vi "CRYGet Changed Acquisition Curve Name.vi"(4 "Change Record Curve Name?":bool, 5 "Origin MR0":string[][](array[string]), 6 "Load?":bool, 7 "Change Channels":bool, 8 "Changed Name Table in":string[][](array[string]), 9 "use ch name":bool, 10 "Old Name":string[][](array[string]), 11 "New Name":string[][](array[string])) -> (0 "Changed Name Table  out":string[][](array[string]))   [LabVIEW 2013]
panel:
  out "Changed Name Table in 2":string[][](array[string])
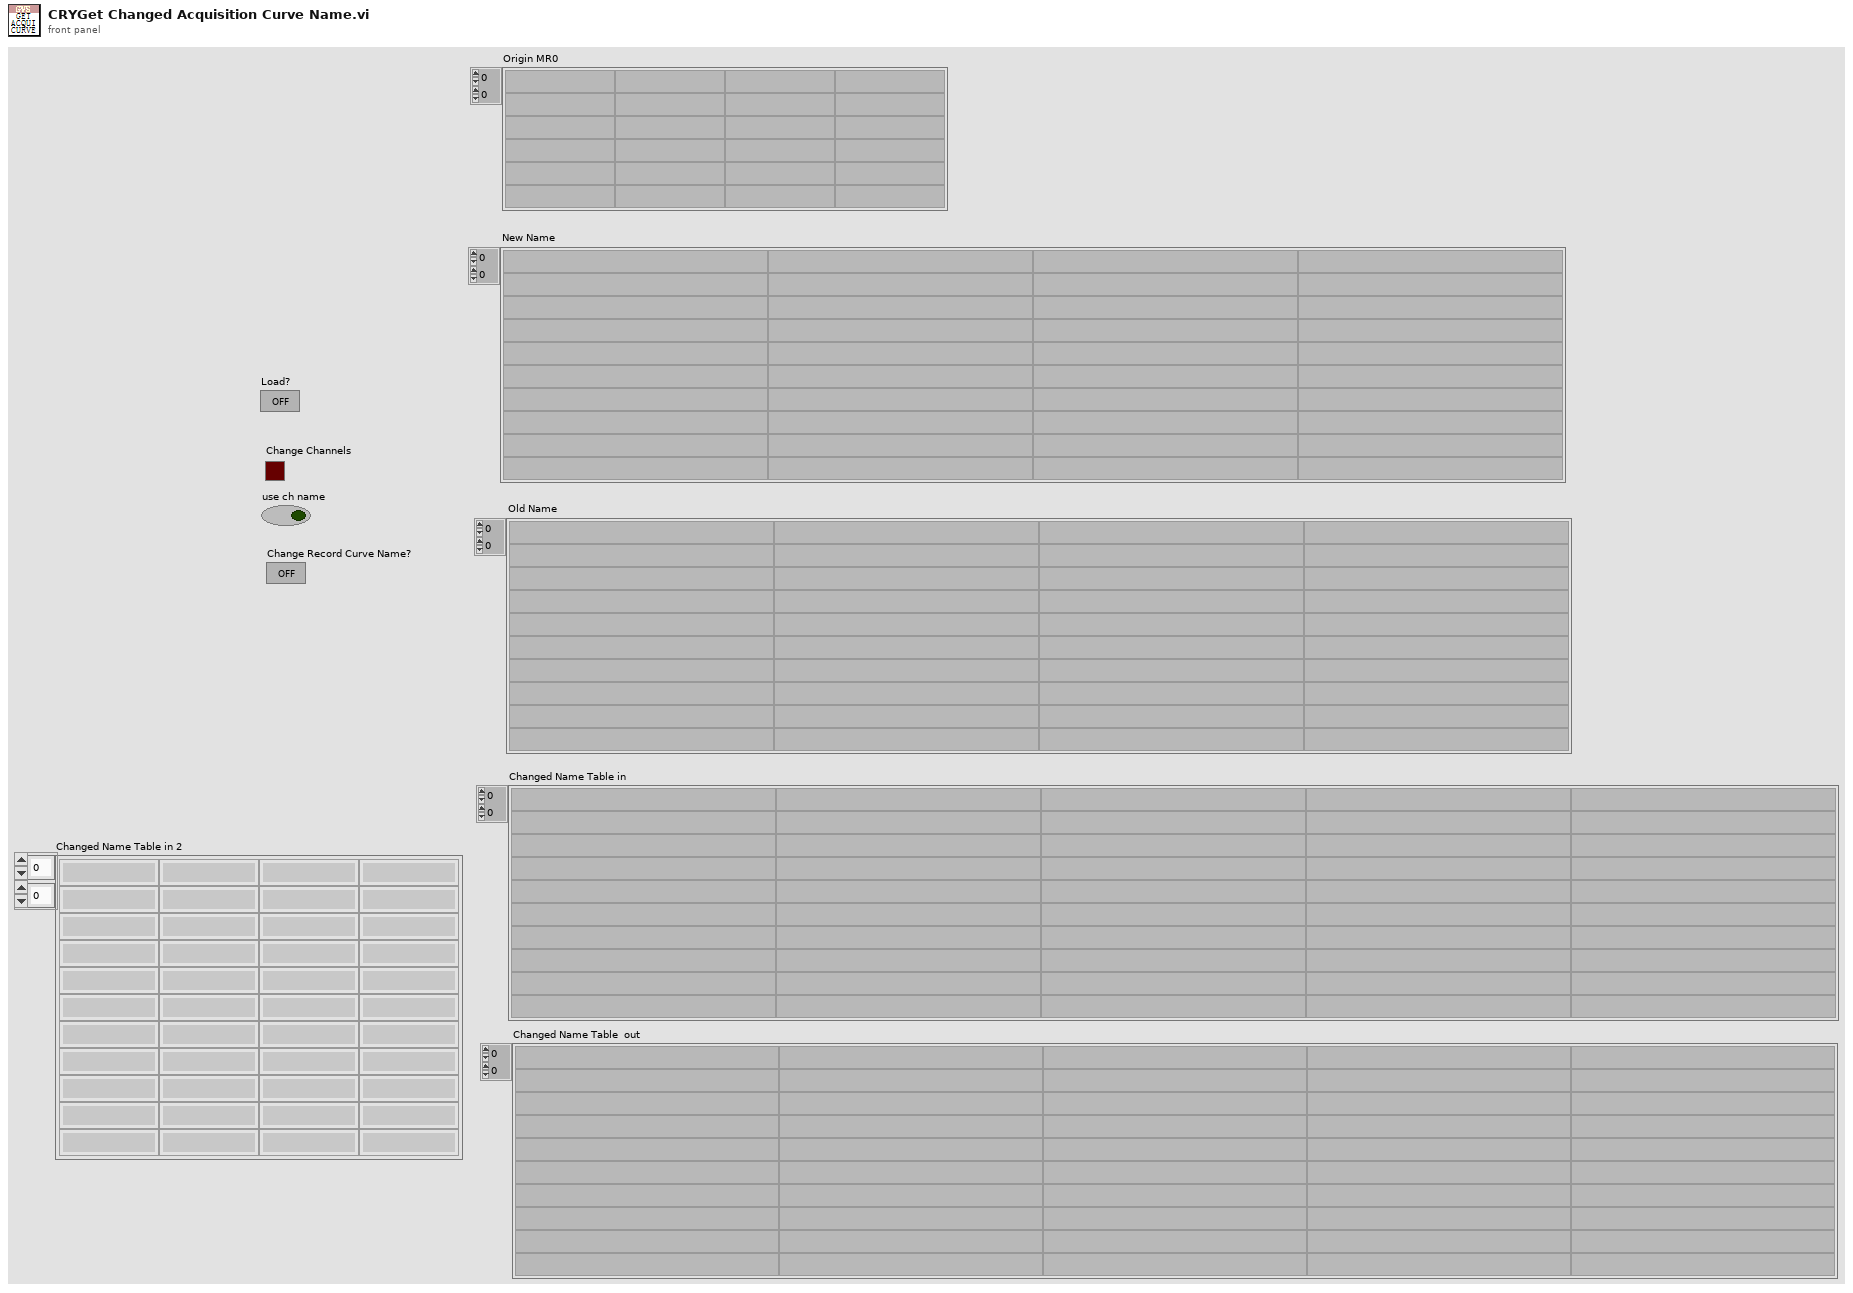
[diagram p1: front panel]
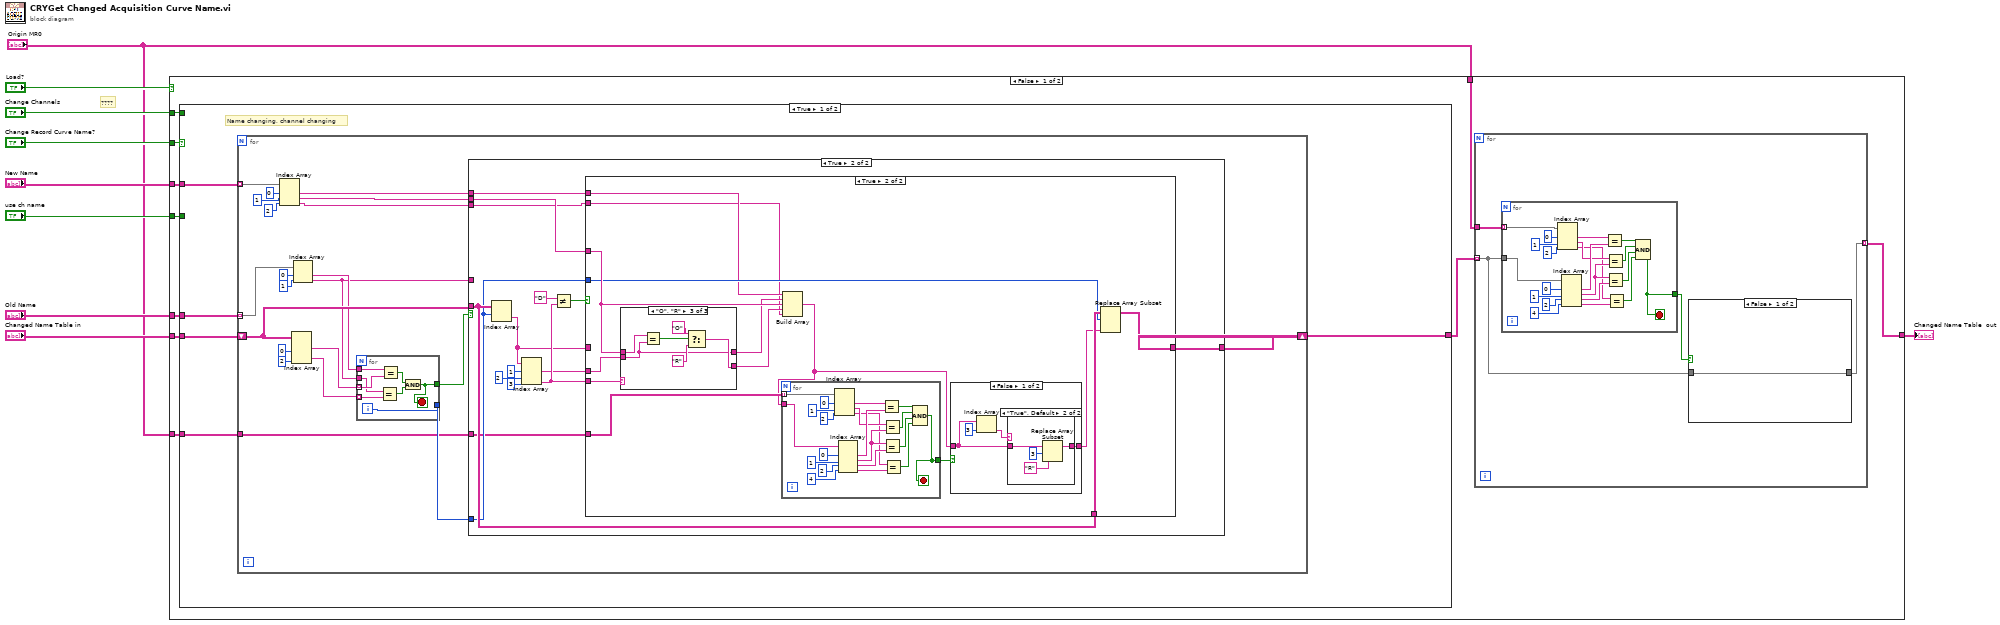
[diagram p0: block diagram]
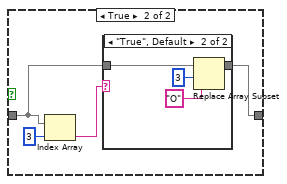
[diagram p2: hidden frame]
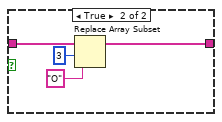
[diagram p7: hidden frame]
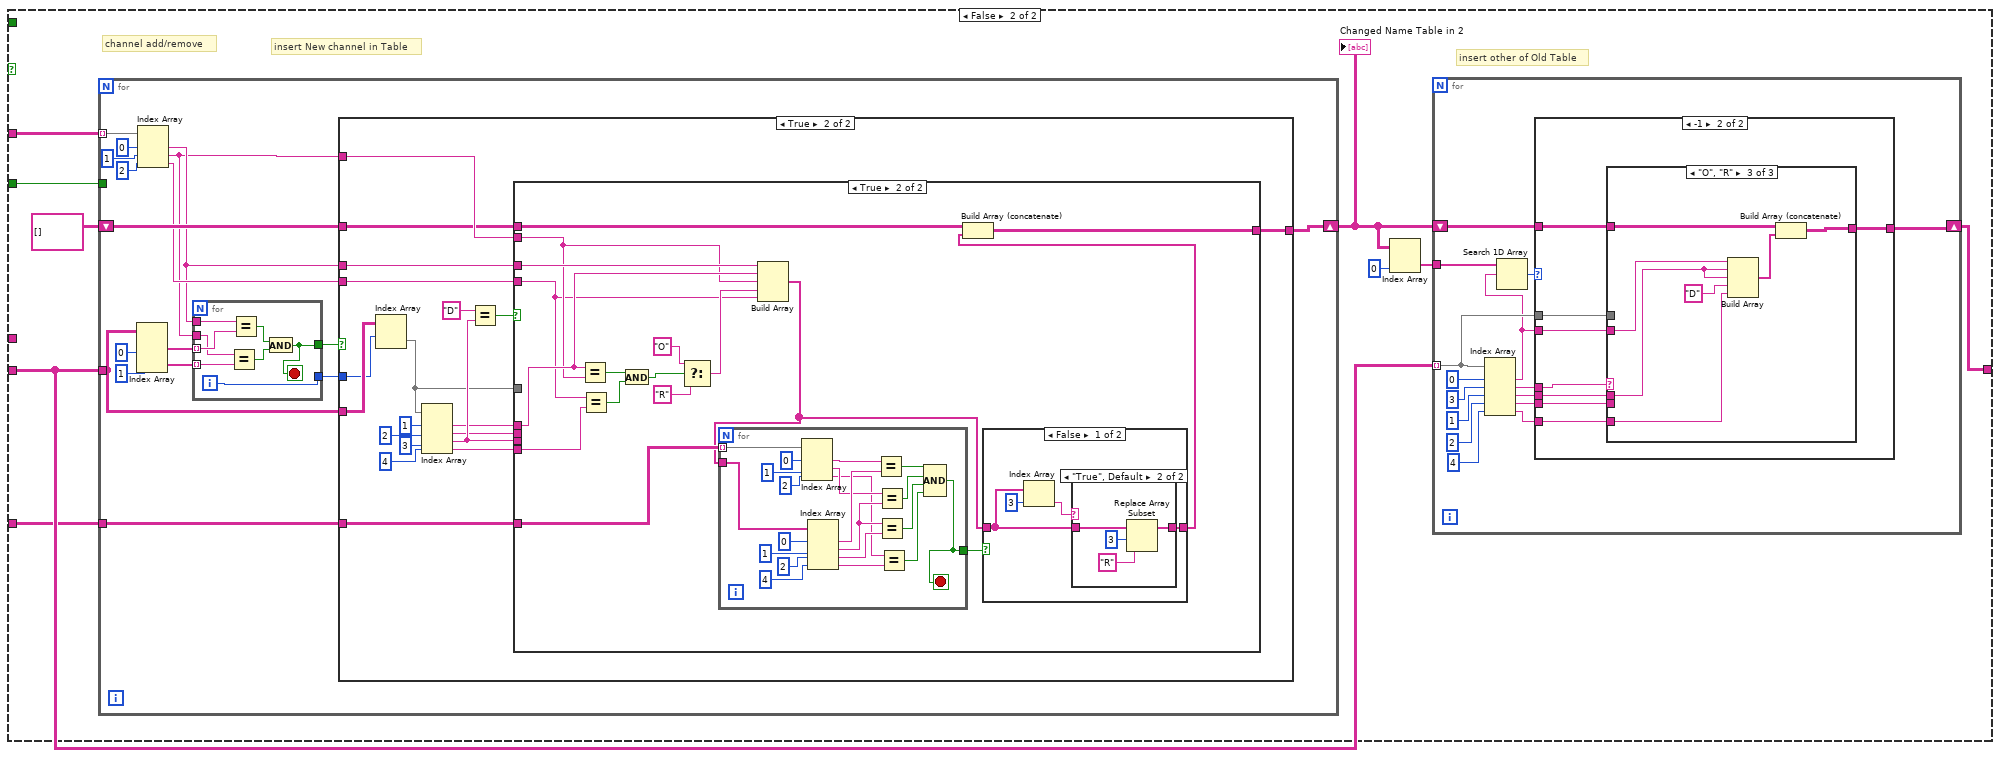
[diagram p10: hidden frame]
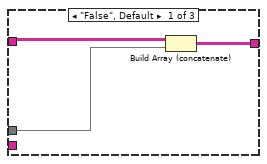
[diagram p12: hidden frame]
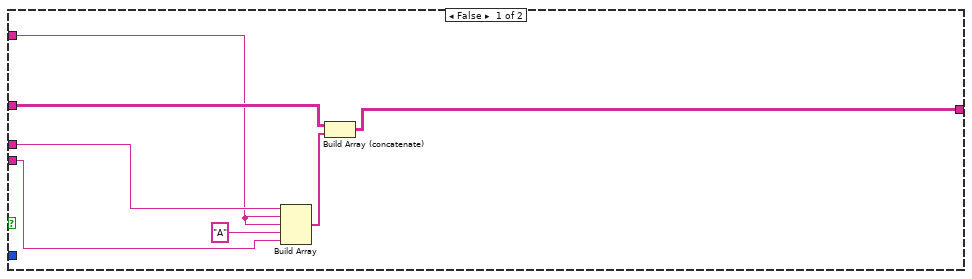
[diagram p14: hidden frame]
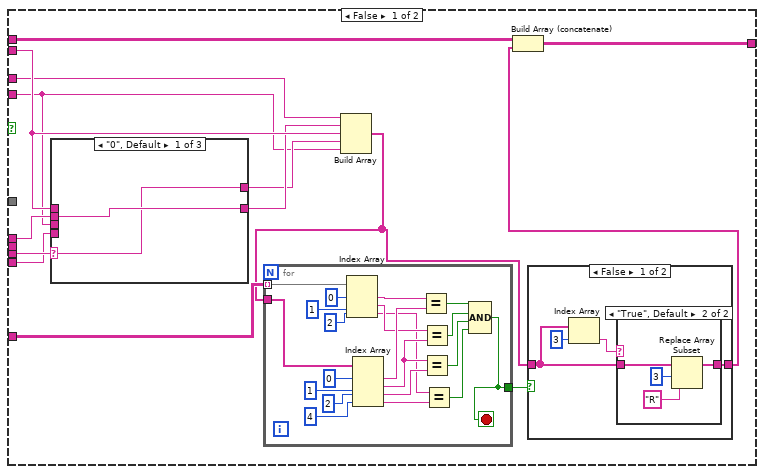
[diagram p15: hidden frame]
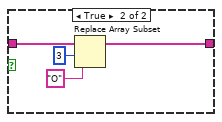
[diagram p17: hidden frame]
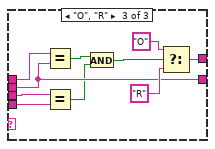
[diagram p19: hidden frame]
diagram:
  # "????"
  n1 = case shown="False" "Load?" {
    tunnel: [w11 w372] -> w9
    tunnel: "Changed Name Table in" -> [w19 _]
    tunnel: "Change Record Curve Name?" -> [w18 _]
    tunnel: "use ch name" -> [w17 _]
    tunnel: "Change Channels" -> [w16 _]
    tunnel: "New Name" -> [w15 w373]
    tunnel: "Old Name" -> [w14 _]
    tunnel: "Origin MR0" -> [w13 _]
    tunnel: "Origin MR0" -> [w10 _]
    frame False {
      n2 = case shown="True" w18 {
        tunnel: [w56 w169] -> w12
        tunnel: w19 -> [w59 w165]
        tunnel: w14 -> [w58 _]
        tunnel: w15 -> [w57 w172]
        tunnel: w17 -> [_ w171]
        tunnel: w16 -> [_ _]
        tunnel: w10 -> [w55 w164]
        frame True {
          # "Name changing, channel changing"
          n3 = for {
            tunnel: w57 -> [w75] mode=indexing
            tunnel: w58 -> [w72] mode=indexing
            shift-right: [w71] -> w56
            shift-left: w59 -> [w80]
            tunnel: w55 -> [w60]
            n4 = Index Array(array=w75, index #1=0 ("index"), index #2=1 ("index"), index #3=2 ("index")) -> (element #1=w70:string, element #2=w78:string, element #3=w61:string)
            n5 = Index Array(array=w80, index (col) #1=0 ("disabled index (col)"), index (col) #2=2 ("index (col)")) -> (element #1=w67:string[], element #2=w68:string[])  [unwired: 2 in]
            n6 = Index Array(array=w72, index #1=0 ("index"), index #2=1 ("index")) -> (element #1=w66:string, element #2=w65:string)
            n7 = for {
              tunnel: w67 -> [w87] mode=indexing
              tunnel: w68 -> [w85] mode=indexing
              tunnel: w66 -> [w88]
              tunnel: w65 -> [w86]
              tunnel: [w82] -> w64
              tunnel: [w81] -> w63
              i -> [w81]
              stop <- w82 stop-if-true
              n8 = Equal?(x=w86, y=w85) -> (x = y?=w83:bool)
              n9 = Equal?(x=w88, y=w87) -> (x = y?=w84:bool)
              n10 = And(x=w84, y=w83) -> (x .and. y?=w82:bool)
            }
            n11 = case shown="True" w64 {
              tunnel: [w89 w95] -> w71
              tunnel: w80 -> [w89 w96]
              tunnel: w78 -> [_ w98]
              tunnel: w65 -> [_ _]
              tunnel: w70 -> [_ w93]
              tunnel: w63 -> [_ w92]
              tunnel: w61 -> [_ w91]
              tunnel: w60 -> [_ w90]
              frame False {
              }
              frame True {
                n12 = Index Array(array=w96, index (row)=w92) -> (element=w97:string[])  [unwired: 1 in]
                n13 = Index Array(array=w97, index #1=1 ("index"), index #2=2 ("index"), index #3=3 ("index")) -> (element #1=w99:string, element #3=w100:string)  [unwired: 1 out]
                n14 = Not Equal?(x="D", y=w100) -> (x != y?=w94:bool)
                n15 = case shown="True" w94 {
                  tunnel: [w105 w113] -> w95
                  tunnel: w97 -> [_ _]
                  tunnel: w100 -> [_ w119]
                  tunnel: w99 -> [_ w116]
                  tunnel: w98 -> [_ w118]
                  tunnel: w96 -> [w105 w114]
                  tunnel: w92 -> [_ w112]
                  tunnel: w93 -> [_ w111]
                  tunnel: w91 -> [_ w110]
                  tunnel: w90 -> [_ w109]
                  frame False {
                  }
                  frame True {
                    n16 = case shown="\"O\", \"R\"" w119 {
                      selector: w119 -> [w154 w156 _]
                      tunnel: w118 -> [_ w157 w159]
                      tunnel: [w155 w157 w158] -> w117
                      tunnel: w116 -> [w155 _ w158]
                      tunnel: [w154 w156 w160] -> w115
                      frame "False", Default {
                      }
                      frame "A" {
                      }
                      frame "O", "R" {
                        n17 = Equal?(x=w159, y=w158) -> (x = y?=w163:bool)
                        n18 = Select(t="O", s=w163, f="R") -> (s? t:f=w160:string)
                      }
                    }
                    n19 = Build Array(w111, w117, w118, w115, w110) -> (w107:string[])
                    n20 = for {
                      tunnel: w109 -> [w150] mode=indexing
                      tunnel: w107 -> [w146]
                      tunnel: [w133] -> w108
                      stop <- w133 stop-if-true
                      n21 = Index Array(array=w150, index #1=0 ("index"), index #2=1 ("index"), index #3=2 ("index")) -> (element #1=w145:string, element #2=w143:string, element #3=w138:string)
                      n22 = Index Array(array=w146, index #1=0 ("index"), index #2=1 ("index"), index #3=2 ("index"), index #4=4 ("index")) -> (element #1=w144:string, element #2=w142:string, element #3=w141:string, element #4=w139:string)
                      n23 = Equal?(x=w145, y=w144) -> (x = y?=w137:bool)
                      n24 = Equal?(x=w143, y=w142) -> (x = y?=w136:bool)
                      n25 = Equal?(x=w142, y=w141) -> (x = y?=w135:bool)
                      n26 = Equal?(x=w138, y=w139) -> (x = y?=w134:bool)
                      n27 = Compound Arithmetic op=AND(w137, w136, w135, w134) -> (w133:bool)
                    }
                    n28 = case shown="False" w108 {
                      tunnel: w107 -> [w122 w132]
                      tunnel: [w123 w129] -> w106
                      frame False {
                        n29 = Index Array(array=w122, index=3) -> (element=w120:string)
                        n30 = case shown="\"True\", Default" w120 {
                          tunnel: [w124 w126] -> w123
                          tunnel: w122 -> [w124 w125]
                          frame "A" {
                          }
                          frame "True", Default {
                            n31 = Replace Array Subset(array=w125, new element="R" ("new element/subarray"), index=3) -> (w126:string[])
                          }
                        }
                      }
                      frame True {
                        n32 = Replace Array Subset(array=w132, new element="O" ("new element/subarray"), index=3) -> (w129:string[])
                      }
                    }
                    n33 = Replace Array Subset(array=w114, new element=w106, index (row)=w112) -> (w113:string[][])  [unwired: 1 in]
                  }
                }
              }
            }
          }
        }
        frame False {
          # "insert other of Old Table"
          # "insert New channel in Table"
          # "channel add/remove"
          n34 = for {
            tunnel: w172 -> [w221] mode=indexing
            shift-right: [w220] -> w168
            shift-left: string[][] [] ("Changed Name Table in") -> [w218]
            tunnel: w171 -> [_]
            tunnel: w165 -> [w219]
            tunnel: w164 -> [w208]
            n35 = Index Array(array=w219, index (col) #1=0 ("disabled index (col)"), index (col) #2=1 ("index (col)")) -> (element #1=w214:string[], element #2=w213:string[])  [unwired: 2 in]
            n36 = Index Array(array=w221, index #1=0 ("index"), index #2=1 ("index"), index #3=2 ("index")) -> (element #1=w212:string, element #2=w211:string, element #3=w216:string)
            n37 = for {
              tunnel: w214 -> [w231] mode=indexing
              tunnel: w213 -> [w229] mode=indexing
              tunnel: w212 -> [w232]
              tunnel: w211 -> [w230]
              tunnel: [w226] -> w210
              tunnel: [w225] -> w209
              i -> [w225]
              stop <- w226 stop-if-true
              n38 = Equal?(x=w230, y=w229) -> (x = y?=w227:bool)
              n39 = Equal?(x=w232, y=w231) -> (x = y?=w228:bool)
              n40 = And(x=w228, y=w227) -> (x .and. y?=w226:bool)
            }
            n41 = case shown="True" w210 {
              tunnel: [w237 w246] -> w220
              tunnel: w219 -> [_ w250]
              tunnel: w211 -> [w234 w252]
              tunnel: w218 -> [w238 w247]
              tunnel: w212 -> [w236 w248]
              tunnel: w216 -> [w233 w244]
              tunnel: w209 -> [_ w243]
              tunnel: w208 -> [_ w240]
              frame False {
                n42 = Build Array(w236, w234, w234, "A" ("element"), w233) -> (w239:string[])
                n43 = Build Array (concatenate)(w238, w239) -> (w237:string[][])
              }
              frame True {
                n44 = Index Array(array=w250, index (row)=w243) -> (element=w251:string[])  [unwired: 1 in]
                n45 = Index Array(array=w251, index #1=1 ("index"), index #2=2 ("index"), index #3=3 ("index"), index #4=4 ("index")) -> (element #1=w253:string, element #2=w245:string, element #3=w254:string, element #4=w241:string)
                n46 = Equal?(x="D", y=w254) -> (x = y?=w249:bool)
                n47 = case shown="True" w249 {
                  tunnel: [w265 w331] -> w246
                  tunnel: w251 -> [_ _]
                  tunnel: w254 -> [w272 _]
                  tunnel: w253 -> [w269 w332]
                  tunnel: w252 -> [w271 w330]
                  tunnel: w248 -> [w267 w336]
                  tunnel: w247 -> [w266 w337]
                  tunnel: w245 -> [_ _]
                  tunnel: w244 -> [w264 w329]
                  tunnel: w241 -> [w263 w325]
                  tunnel: w240 -> [w262 w324]
                  frame False {
                    n48 = case shown="\"0\", Default" w272 {
                      selector: w272 -> [w307 w309 _]
                      tunnel: w271 -> [_ w310 w317]
                      tunnel: [w308 w310 w316] -> w270
                      tunnel: w269 -> [w308 _ w316]
                      tunnel: [w307 w309 w318] -> w268
                      tunnel: w264 -> [_ _ w312]
                      tunnel: w263 -> [_ _ w311]
                      frame "0", Default {
                      }
                      frame "A" {
                      }
                      frame "O", "R" {
                        n49 = Equal?(x=w317, y=w316) -> (x = y?=w314:bool)
                        n50 = Equal?(x=w312, y=w311) -> (x = y?=w315:bool)
                        n51 = And(x=w314, y=w315) -> (x .and. y?=w313:bool)
                        n52 = Select(t="O", s=w313, f="R") -> (s? t:f=w318:string)
                      }
                    }
                    n53 = Build Array(w267, w270, w271, w268, w264) -> (w260:string[])
                    n54 = for {
                      tunnel: w262 -> [w303] mode=indexing
                      tunnel: w260 -> [w299]
                      tunnel: [w286] -> w261
                      stop <- w286 stop-if-true
                      n55 = Index Array(array=w303, index #1=0 ("index"), index #2=1 ("index"), index #3=2 ("index")) -> (element #1=w298:string, element #2=w296:string, element #3=w291:string)
                      n56 = Index Array(array=w299, index #1=0 ("index"), index #2=1 ("index"), index #3=2 ("index"), index #4=4 ("index")) -> (element #1=w297:string, element #2=w295:string, element #3=w294:string, element #4=w292:string)
                      n57 = Equal?(x=w298, y=w297) -> (x = y?=w290:bool)
                      n58 = Equal?(x=w296, y=w295) -> (x = y?=w289:bool)
                      n59 = Equal?(x=w295, y=w294) -> (x = y?=w288:bool)
                      n60 = Equal?(x=w291, y=w292) -> (x = y?=w287:bool)
                      n61 = Compound Arithmetic op=AND(w290, w289, w288, w287) -> (w286:bool)
                    }
                    n62 = case shown="False" w261 {
                      tunnel: w260 -> [w275 w285]
                      tunnel: [w276 w282] -> w259
                      frame False {
                        n63 = Index Array(array=w275, index=3) -> (element=w273:string)
                        n64 = case shown="\"True\", Default" w273 {
                          tunnel: [w277 w279] -> w276
                          tunnel: w275 -> [w277 w278]
                          frame "A" {
                          }
                          frame "True", Default {
                            n65 = Replace Array Subset(array=w278, new element="R" ("new element/subarray"), index=3) -> (w279:string[])
                          }
                        }
                      }
                      frame True {
                        n66 = Replace Array Subset(array=w285, new element="O" ("new element/subarray"), index=3) -> (w282:string[])
                      }
                    }
                    n67 = Build Array (concatenate)(w266, w259) -> (w265:string[][])
                  }
                  frame True {
                    n68 = Equal?(x=w332, y=w330) -> (x = y?=w328:bool)
                    n69 = Equal?(x=w329, y=w325) -> (x = y?=w326:bool)
                    n70 = And(x=w328, y=w326) -> (x .and. y?=w327:bool)
                    n71 = Select(t="O" ("x"), s=w327, f="R") -> (s? t:f=w333:string)
                    n72 = Build Array(w336, w332, w330, w333, w329) -> (w322:string[])
                    n73 = for {
                      tunnel: w324 -> [w368] mode=indexing
                      tunnel: w322 -> [w364]
                      tunnel: [w351] -> w323
                      stop <- w351 stop-if-true
                      n74 = Index Array(array=w368, index #1=0 ("index"), index #2=1 ("index"), index #3=2 ("index")) -> (element #1=w363:string, element #2=w361:string, element #3=w356:string)
                      n75 = Index Array(array=w364, index #1=0 ("index"), index #2=1 ("index"), index #3=2 ("index"), index #4=4 ("index")) -> (element #1=w362:string, element #2=w360:string, element #3=w359:string, element #4=w357:string)
                      n76 = Equal?(x=w363, y=w362) -> (x = y?=w355:bool)
                      n77 = Equal?(x=w361, y=w360) -> (x = y?=w354:bool)
                      n78 = Equal?(x=w360, y=w359) -> (x = y?=w353:bool)
                      n79 = Equal?(x=w356, y=w357) -> (x = y?=w352:bool)
                      n80 = Compound Arithmetic op=AND(w355, w354, w353, w352) -> (w351:bool)
                    }
                    n81 = case shown="False" w323 {
                      tunnel: w322 -> [w340 w350]
                      tunnel: [w341 w347] -> w321
                      frame False {
                        n82 = Index Array(array=w340, index=3) -> (element=w338:string)
                        n83 = case shown="\"True\", Default" w338 {
                          tunnel: [w342 w344] -> w341
                          tunnel: w340 -> [w342 w343]
                          frame "A" {
                          }
                          frame "True", Default {
                            n84 = Replace Array Subset(array=w343, new element="R" ("new element/subarray"), index=3) -> (w344:string[])
                          }
                        }
                      }
                      frame True {
                        n85 = Replace Array Subset(array=w350, new element="O" ("new element/subarray"), index=3) -> (w347:string[])
                      }
                    }
                    n86 = Build Array (concatenate)(w337, w321) -> (w331:string[][])
                  }
                }
              }
            }
          }
          "Changed Name Table in 2" <- w168
          n87 = Index Array(array=w168, index (col)=0 ("disabled index (col)")) -> (element=w166:string[])  [unwired: 1 in]
          n88 = for {
            shift-right: [w180] -> w169
            shift-left: w168 -> [w185]
            tunnel: w166 -> [w187]
            tunnel: w165 -> [w183] mode=indexing
            n89 = Index Array(array=w183, index #1=0 ("index"), index #2=3 ("index"), index #3=1 ("index"), index #4=2 ("index"), index #5=4 ("index")) -> (element #1=w177:string, element #2=w181:string, element #3=w176:string, element #4=w175:string, element #5=w173:string)
            n90 = Search 1D Array(1D array=w187, element=w177) -> (index of element=w186:i32)  [unwired: 1 in]
            n91 = case shown="-1" w186 {
              tunnel: w185 -> [w188 w196]
              tunnel: w183 -> [_ w194]
              tunnel: w181 -> [_ w193]
              tunnel: [w188 w195] -> w180
              tunnel: w177 -> [_ w192]
              tunnel: w176 -> [_ w191]
              tunnel: w175 -> [_ w190]
              tunnel: w173 -> [_ w189]
              frame 0, Default {
              }
              frame -1 {
                n92 = case shown="\"O\", \"R\"" w193 {
                  tunnel: w196 -> [w199 w200 w207]
                  tunnel: [w198 w200 w206] -> w195
                  tunnel: w194 -> [w197 _ _]
                  tunnel: w192 -> [_ _ w205]
                  tunnel: w191 -> [_ _ w202]
                  tunnel: w190 -> [_ _ _]
                  tunnel: w189 -> [_ _ w201]
                  frame "False", Default {
                    n93 = Build Array (concatenate)(w199, w197) -> (w198:string[][])
                  }
                  frame "A" {
                  }
                  frame "O", "R" {
                    n94 = Build Array(w205, w202, w202, "D" ("Custom Curve Names"), w201) -> (w204:string[])
                    n95 = Build Array (concatenate)(w207, w204) -> (w206:string[][])
                  }
                }
              }
            }
          }
        }
      }
      n96 = for {
        tunnel: w13 -> [w23]
        tunnel: w12 -> [w22] mode=indexing
        tunnel: [w20] -> w11 mode=indexing
        n97 = for {
          tunnel: w23 -> [w51] mode=indexing
          tunnel: w22 -> [w47]
          tunnel: [w34] -> w21
          stop <- w34 stop-if-true
          n98 = Index Array(array=w51, index #1=0 ("index"), index #2=1 ("index"), index #3=2 ("index")) -> (element #1=w46:string, element #2=w44:string, element #3=w39:string)
          n99 = Index Array(array=w47, index #1=0 ("index"), index #2=1 ("index"), index #3=2 ("index"), index #4=4 ("index")) -> (element #1=w45:string, element #2=w43:string, element #3=w42:string, element #4=w40:string)
          n100 = Equal?(x=w46, y=w45) -> (x = y?=w38:bool)
          n101 = Equal?(x=w44, y=w43) -> (x = y?=w37:bool)
          n102 = Equal?(x=w43, y=w42) -> (x = y?=w36:bool)
          n103 = Equal?(x=w39, y=w40) -> (x = y?=w35:bool)
          n104 = Compound Arithmetic op=AND(w38, w37, w36, w35) -> (w34:bool)
        }
        n105 = case shown="False" w21 {
          tunnel: w22 -> [w24 w27]
          tunnel: [w24 w28] -> w20
          frame False {
          }
          frame True {
            n106 = Index Array(array=w27, index=3) -> (element=w25:string)
            n107 = case shown="\"True\", Default" w25 {
              tunnel: w27 -> [w29 w33]
              tunnel: [w29 w30] -> w28
              frame "D" {
              }
              frame "True", Default {
                n108 = Replace Array Subset(array=w33, new element="O" ("new element/subarray"), index=3) -> (w30:string[])
              }
            }
          }
        }
      }
    }
    frame True {
      n109 = for {
        tunnel: w373 -> [w381] mode=indexing
        tunnel: [w382] -> w372 mode=indexing
        n110 = Index Array(array=w381, index #1=0 ("index"), index #2=1 ("index"), index #3=2 ("index")) -> (element #1=w377:string, element #2=w374:string, element #3=w376:string)
        n111 = Build Array(w377, w374, w374, "O", w376) -> (w382:string[])
      }
    }
  }
  "Changed Name Table  out" <- w9
